vi "Read N.vi"(9 "ForLoop in":refnum<class "ForLoop.lvclass">) -> (3 "ForLoop out":refnum<class "ForLoop.lvclass">, 4 "N":refnum<class "Tunnel.lvclass">)   [LabVIEW 2014, in "ForLoop.lvclass"]
uses:
  ForLoop.lvclass
  Tunnel/Tunnel.lvclass
  ForLoop.lvclass/ForLoop.ctl
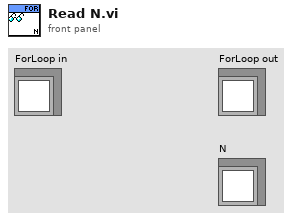
[diagram p1: front panel]
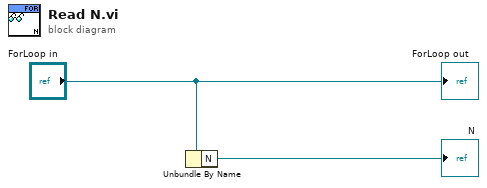
[diagram p0: block diagram]
diagram:
  n1 = Unbundle By Name("ForLoop in") -> ("N"=→"N":refnum<class "Tunnel.lvclass">)
  "ForLoop out" <- "ForLoop in"
